vi "close_current_dataset.vi"(8 "error in (no error)":errorcluster, 11 "pcfs_hdf5_log in":refnum<class "pcfs_hdf5_log.lvclass">) -> (0 "error out":errorcluster, 3 "pcfs_hdf5_log out":refnum<class "pcfs_hdf5_log.lvclass">)   [LabVIEW 2015, in "pcfs_hdf5_log.lvclass"]
uses:
  pcfs_hdf5_log.lvclass
  pcfs_hdf5_log.lvclass/pcfs_hdf5_log.ctl
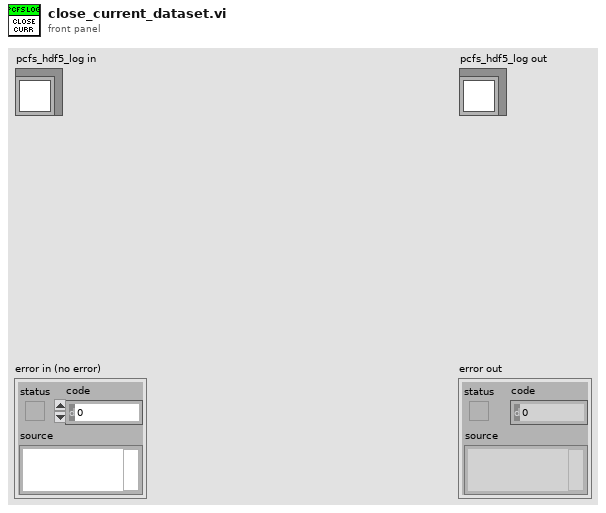
[diagram p1: front panel]
types:
  T1 = typedef "hpanel_acq_modes.ctl" = u16
  T2 = typedef "HDF5 Ref.ctl" = refnum<k1>
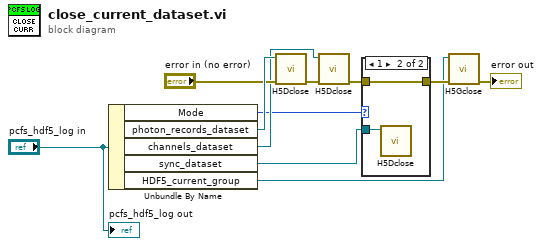
[diagram p0: block diagram]
diagram:
  n1 = Unbundle By Name("pcfs_hdf5_log in") -> ("Mode"=w6:T1, "photon_records_dataset"=w11:T2, "channels_dataset"=w9:T2, "sync_dataset"=w8:T2, "HDF5_current_group"=w3:T2)
  n2 = call <vilib>:"H5Dclose.vi"("error in (no error)"="error in (no error)", "HDF5 Dataset Ref"=w11) -> ("error out"=w7:errorcluster)  [unwired: 7 in]
  n3 = call <vilib>:"H5Dclose.vi"("error in (no error)"=w7, "HDF5 Dataset Ref"=w9) -> ("error out"=w5:errorcluster)  [unwired: 7 in]
  n4 = case shown="1" w6 {
    tunnel: w8 -> [_ w14]
    tunnel: w5 -> [w12 w13]
    tunnel: [w12 w13] -> w4
    frame 0, Default {
    }
    frame 1 {
      n5 = call <vilib>:"H5Dclose.vi"("HDF5 Dataset Ref"=w14) -> ()  [unwired: 8 in, 1 out]
    }
  }
  n6 = call <vilib>:"H5Gclose.vi"("error in (no error)"=w4, "HDF5 Group Ref"=w3) -> ("error out"=→"error out":errorcluster)  [unwired: 7 in]
  "pcfs_hdf5_log out" <- "pcfs_hdf5_log in"
